vi "EncoderTDMS_Path.vi"(8 "error in (no error)":errorcluster, 9 "Operation (Read)":enum16{"Write", "Read"}(ring)=enum."Read", 11 "PathIn":path) -> (0 "error out":errorcluster, 3 "Path Out":path)   [LabVIEW 2020]
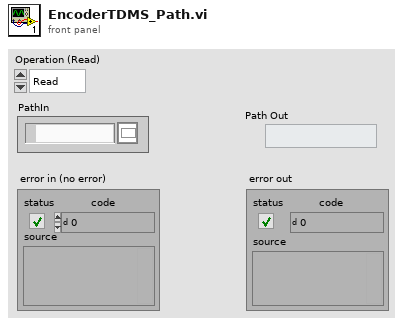
[diagram p1: front panel]
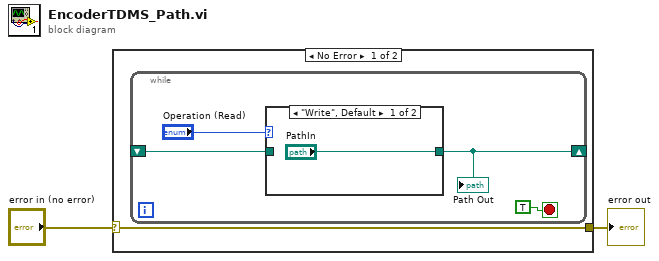
[diagram p0: block diagram]
diagram:
  n1 = case shown="No Error" "error in (no error)" {
    selector: "error in (no error)" -> [w3 w10]
    tunnel: [w3 w10] -> w1
    frame No Error {
      n2 = while {
        shift-right: [w4] -> _
        shift-left: _ -> [w5]
        stop <- TRUE stop-if-true
        n3 = case shown="\"Write\", Default" "Operation (Read)" {
          tunnel: ["PathIn" w9] -> w4
          tunnel: w5 -> [_ w9]
          frame "Write", Default {
          }
          frame "Read" {
          }
        }
        "Path Out" <- w4
      }
    }
    frame Error {
    }
  }
  "error out" <- w1
